vi "AWS-S3-InitializeClient.vi"(5 "Access Key":string, 7 "Secret Key":string, 11 "error in":errorcluster) -> (4 "Mini AWS S3 API":refnum<class "AWS-S3-MiniAPI.lvclass">, 15 "error out":errorcluster)   [LabVIEW 2012, in "AWS-S3-MiniAPI.lvclass"]
uses:
  AWS-S3-MiniAPI.lvclass
  C:/Users/Jack/cla-2013-deployment-automation-and-release-engineering-in-labview/Deployment/AWS-SDK/AWSSDK.dll
  AWS-SDK/AWSSDK.dll
  AWS-S3-MiniAPI.lvclass/AWS-S3-MiniAPI.ctl
panel:
  # "Inputs"
  # "Outputs"
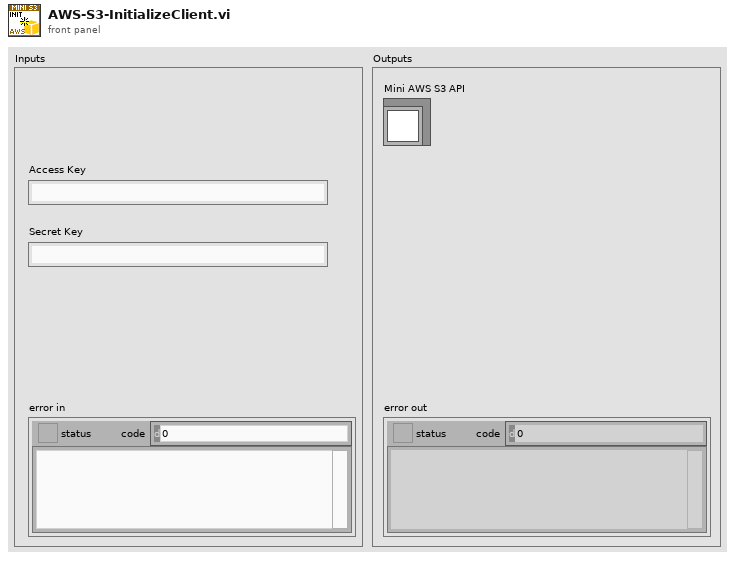
[diagram p1: front panel]
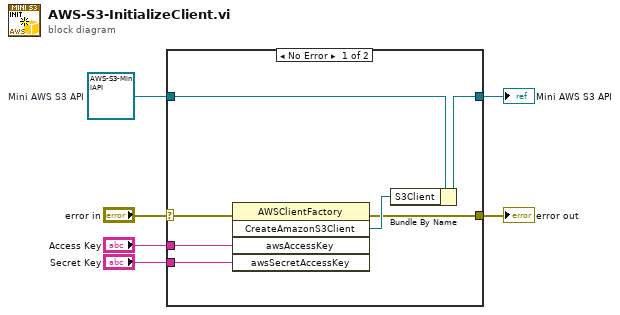
[diagram p0: block diagram]
diagram:
  w5 = refnum<class "AWS-S3-MiniAPI.lvclass"> refnum  # Mini AWS S3 API
  n1 = case shown="No Error" "error in" {
    selector: "error in" -> [w8 w15]
    tunnel: [w7 w15] -> w6
    tunnel: [w12 w14] -> w4
    tunnel: w5 -> [w13 w14]
    tunnel: "Access Key" -> [w10 _]
    tunnel: "Secret Key" -> [w9 _]
    frame No Error {
      n2 = invoke class="AWSClientFactory" method="CreateAmazonS3Client"(error in=w8, "awsAccessKey"=w10, "awsSecretAccessKey"=w9) -> (error out=w7:errorcluster, "CreateAmazonS3Client"=w11:refnum<k24>)  [unwired: 2 in, 3 out]
      n3 = Bundle By Name(cluster=w13, "S3Client"=w11) -> (w12:refnum<class "AWS-S3-MiniAPI.lvclass">)
    }
    frame Error {
    }
  }
  "error out" <- w6
  "Mini AWS S3 API" <- w4
